vi "Tap Example.vi"() -> ()   [LabVIEW 2023, in "GettingStarted_Tap_148X_Host.lvlib"]
uses:
  GettingStarted_Tap_148X_Host.lvlib
  Acq/GettingStarted_Acq_148X_Host.lvlib
  <instrlib>/FlexRIO/API/Host/v1/NI FlexRIO API v1.lvlib
  Common/GettingStarted_Common_148X_Host.lvlib
  <vilib>/vision/Image Controls.llb/IMAQ Image.ctl
  Common/Types/Packet Table.ctl
  <vilib>/Utility/miscctls.llb/LVRowAndColumnUnsignedTypeDef.ctl
  <vilib>/rvi/interface/nirviCloseFPGA/nirviCloseFPGA.xnode
  <vilib>/FPGAPlugInAG/Dynamic/niLvFpga_Close_Dynamic.vi
  <instrlib>/FlexRIO/API/Host/v1/NI FlexRIO/API/Wait for PoC Safe to Disconnect Channels Array.vi
  <instrlib>/FlexRIO/CSI-2/v2/Common/Types/LLP Data Type.ctl
  <instrlib>/FlexRIO/CSI-2/v2/Common/NI CSI-2 API Common v2.lvlib
  <vilib>/userDefined/Silver/nirio_resource_slv.ctl
  Acq/Types/CSI-2 Data Source.ctl
  <instrlib>/FlexRIO/CSI-2/v2/FPGA/Types/Timestamp ID.ctl
  <instrlib>/FlexRIO/CSI-2/v2/FPGA/NI CSI-2 API FPGA v2.lvlib
  Common/Types/GPIO Filter.ctl
  <instrlib>/FlexRIO/CSI-2/v2/FPGA/Types/GPIO Bank.ctl
  FPGA/Common/Types/SerDes Identifier.ctl
  FPGA/Common/GettingStarted_Common_148X_FPGA.lvlib
  Common/Types/GPIO Route Direction.ctl
  Common/Types/GPIO Route Line.ctl
  Common/Types/GPIO Route Configuration.ctl
  <instrlib>/FlexRIO/CSI-2/v2/FPGA/Types/Display Parameters.ctl
  Common/Types/RAW Interpretation for Display.ctl
  Types/Serial Channel Tap Pair.ctl
  Types/Serial Channel Tap Configuration.ctl
panel:
  out "Acquisition Stopped":bool
  in  "Acquired Serial Input Channel Data":T1(tab)
  out "Source Rate (fps)(1st Display)":dbl
  out "Update Rate (fps)(1st Display)":dbl
  in  "Serial Channel (1st Display)":fxp<+,3,3>
  out "1st channel display":T2(plugin-control)
  out "Source Rate (fps)(2nd Display)":dbl
  out "Update Rate (fps)(2nd Display)":dbl
  out "2nd channel display":T2(plugin-control)
  in  "Serial Channel (2nd Display)":fxp<+,3,3>
  out "Acquired Packets (1st Channel)":T3
  out "Packets Logged (1st Channel)":i64
  out "Bytes Acquired (1st Channel)":i64 format="%#.6p"
  out "Acquired Packets (2nd Channel)":T3
  out "Packets Logged (2nd Channel)":i64
  out "Bytes Acquired (2nd Channel)":i64 format="%#.6p"
  out "I2C Timestamps":T3
  out "Error Parsing GPIO Timestamps":bool
  out "GPIO Timestamps Waveform":digitalwaveform[](graph)
  in  "Configuration":T4(tab)
  in  "Log Packets to Disk":bool
  in  "Display Acquired Images":bool=TRUE
  in  "RIO Device":T5
  in  "Bitfile Path":path
  in  "TDMS File Directory":path
  in  "Log I2C to Disk":bool
  in  "Log GPIO to Disk":bool
  in  "Logged Packets to Display":i64=1400
  in  "Channel Configurations":T6[](array[typedef])=[{"Serial Channel Tap Pair"={"input"="SI0", "output"="SO0"}, "FPGA Display Parameters"={"virtual channel"=0.0, "payload data type"=enum."RAW 12", "frame skip count"=0, "line skip count"=0, "pixel skip count"=0.0}, "RAW Display Parameters"={"Interpretation"=enum."Bayer", "Bayer Parameters"={"Pattern"=3, "Algorithm"=0, "Red Gain"=1.0, "Green Gain"=1.0, "Blue Gain"=1.0}}}] {"RAW Display Parameters"."Bayer Parameters"."Blue Gain" min=0.0 max=3.99 step=0.1 format="%_4g"; "RAW Display Parameters"."Bayer Parameters"."Green Gain" min=0.0 max=3.99 step=0.1 format="%_4g"; "RAW Display Parameters"."Bayer Parameters"."Red Gain" min=0.0 max=3.99 step=0.1 format="%_4g"; "RAW Display Parameters"."Bayer Parameters"."Algorithm" items=["Bilinear", "VNG"]; "RAW Display Parameters"."Bayer Parameters"."Pattern" items=["GB", "GR", "BG", "RG"]}
  in  "CSI-2 Data Source":T11=1 items=["Raw", "Corrected"]
  in  "Deserializer (Input) Configuration Script":path
  in  "Serializer (Output) Configuration Script":path
  in  "Continuous Acquisition":bool=TRUE
  in  "Acquisition Duration (s)":dbl=1.0 format="%#_13g"
  in  "Enable First and Last Packet Select":bool=TRUE
  in  "Stop Timeout (s)":dbl=1.0
  in  "First Packet Data Type Select":T9
  in  "Last Packet Data Type Select":T9=enum."Frame End"
  in  "Data Type Filter":T9[](array[typedef])
  in  "Virtual Channel Filter":fxp<+,4,4>[](array[numeric])
  in  "Invert Data Type Filter":bool
  in  "Invert Virtual Channel Filter":bool
  in  "Serial Input Active Lane Count":i32(ring)=4 items=["1 Lane"=1, "2 Lanes"=2, "4 Lanes"=4]
  out "Actual Serial Output Data Rate (bps)":dbl=-1.0 format="%#_6p"
  in  "Requested Serial Ouptut Data Rate (bps)":dbl=-1.0 format="%#_6p"
  in  "Serial Output Active Lane Count":i32(ring)=4 items=["1 Lane"=1, "2 Lanes"=2, "4 Lanes"=4]
  in  "Power Over Coax Source":i32(ring) items=["None", "Internal", "Auxiliary"]
  in  "Power Over Coax Sink":i32(ring) items=["None"=0, "Auxiliary"=2]
  in  "Serial Input Reference Clock Frequency (Hz)":dbl=25000000.0 format="%#_6p"
  in  "Serial Output Reference Clock Frequency (Hz)":dbl=25000000.0 format="%#_6p"
  in  "timestamp filter":T12[](array[typedef])
  in  "GPIO Bank Output Enable":T13
  in  "GPIO Routes":T14[](array[typedef]) {"Serial Channel" max=3 step=1}
  in  "GPIO Bank Select":T17
  in  "Update GPIO Output":bool
  in  "GPIO Bank Output":T13
  out "GPIO Bank Read":T13
  in  "GPIO to Display":T18[](array[typedef])
  out "Acquisition Duration (s)":dbl format="%.1f"
  out "Waiting for Sensor Setup":bool
  in  "Sensor Setup Complete":bool
  out "Power Over Coax Sink In Range":bool[](array[boolean])
  out "Acquisition In Progress":bool
  out "Power Over Coax Voltage (V)":dbl[](array[numeric]) format="%#.2pV"
  out "Power Over Coax Current (A)":dbl[](array[numeric]) format="%#.2pA"
  out "Power Over Coax Source In Range":bool[](array[boolean])
  in  "Stop Acquisition":bool
  out "Error Out":errorcluster
  # "Overview: Configure a tap acquisition for a CSI-2 sensor. Forward acquired CSI-2 data from the serial input channel to the paired serial output channel.\nBridge I2C communication between the paired serial output channel and serial input channel. Transfer the acquired data and timestamps to disk.\nInstructions: Visit https://ni.com/r/automotive-camera-module-ref for tutorials and reference material on using this example with the PXIe-148X."
  # "Configuration Settings"
  # "Data Output"
  # "* For additional packet viewing capability, use GettingStarted_Common_148X_Host.lvlib->TDMS File Viewer.vi"
  # "* For additional packet viewing capability, use GettingStarted_Common_148X_Host.lvlib->TDMS File Viewer.vi"
  # "Resource Configuration"
  # "Output Configuration"
  # "Channel Configuration"
  # "Acquisition Configuration"
  # "First and Last Packet Select Configuration"
  # "Packet Filter Configuration"
  # "Power Over Coax Configuration"
  # "Clocking Configuration"
  # "CSI-2 Output Configuration"
  # "Use -1 to request the default data rate"
  # "I2C Timestamp Configuration"
  # "The timestamp filters listed correspond to the I2C traffic for a specific serial channel:\n\nUser24 = SI0\nUser25 = SI1\nUser26 = SI2\nUser27 = SI3"
  # "GPIO Display Configuration"
  # "GPIO Bank Read / Write Configuration"
  # "GPIO Routing Configuration"
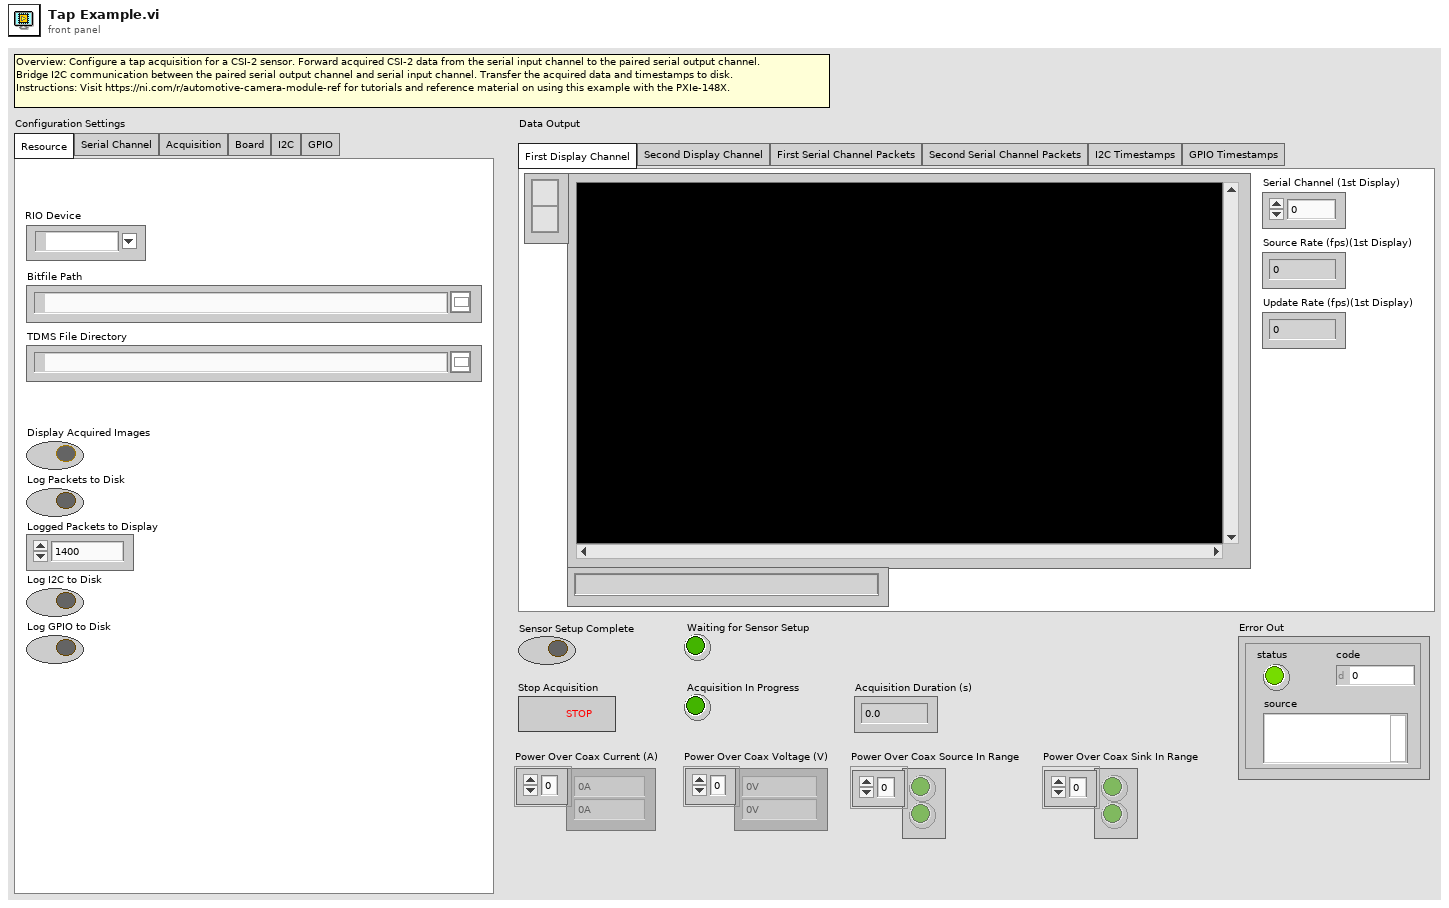
[diagram p1: front panel]
types:
  T1 = enum32{"First Display Channel", "Second Display Channel", "First Serial Channel Packets", "Second Serial Channel Packets", "I2C Timestamps", "GPIO Timestamps"}
  T2 = typedef "IMAQ Image.ctl" = refnum<image>
  T3 = typedef "GettingStarted_Common_148X_Host.lvlib/Packet Table.ctl" = string[][]
  T4 = enum32{"Resource", "Serial Channel", "Acquisition", "Board", "I2C", "GPIO"}
  T5 = typedef "nirio_resource_slv.ctl" = tag
  T6 = typedef "GettingStarted_Tap_148X_Host.lvlib/Serial Channel Tap Configuration.ctl" = cluster{"Serial Channel Tap Pair":T7, "FPGA Display Parameters":T8, "RAW Display Parameters":cluster{"Interpretation":T10, "Bayer Parameters":cluster{"Pattern":i32, "Algorithm":i32, "Red Gain":dbl, "Green Gain":dbl, "Blue Gain":dbl}}}
  T7 = typedef "GettingStarted_Tap_148X_Host.lvlib/Serial Channel Tap Pair.ctl" = cluster{"input":string, "output":string}
  T8 = typedef "NI CSI-2 API FPGA v2.lvlib/Display Parameters.ctl" = cluster{"virtual channel":fxp<+,4,4>, "payload data type":T9, "frame skip count":u16, "line skip count":u8, "pixel skip count":fxp<+,5,5>}
  T9 = typedef "NI CSI-2 API Common v2.lvlib/LLP Data Type.ctl" = enum8{"Frame Start", "Frame End", "Line Start", "Line End", "End of Transmission", "Reserved 0", "Reserved 1", "Reserved 2", "Generic Short Packet 1", "Generic Short Packet 2", "Generic Short Packet 3", "Generic Short Packet 4", "Generic Short Packet 5", "Generic Short Packet 6", "Generic Short Packet 7", "Generic Short Packet 8", "Null", "Blanking Data", "Embedded 8-bit non Image Data", "Generic Long Packet 1", "Generic Long Packet 2", "Generic Long Packet 3", "Generic Long Packet 4", "Reserved 3", "YUV420 8-bit", "YUV420 10-bit", "Legacy YUV420 8-bit", "Reserved 4", "YUV420 8-bit Chroma Shifted", "YUV420 10-bit Chroma Shifted", "YUV422 8-bit", "YUV422 10-bit", "RGB444", "RGB555", "RGB565", "RGB666", "RGB888", "Reserved 5", "Reserved 6", "RAW 24", "RAW 6", "RAW 7", "RAW 8", "RAW 10", "RAW 12", "RAW 14", "RAW 16", "RAW 20", "User Defined 8-bit Data 1", "User Defined 8-bit Data 2", "User Defined 8-bit Data 3", "User Defined 8-bit Data 4", "User Defined 8-bit Data 5", "User Defined 8-bit Data 6", "User Defined 8-bit Data 7", "User Defined 8-bit Data 8", "USL Command", "Reserved 7", "Reserved 8", "Reserved 9", "Reserved 10", "Reserved 11", "Reserved 12", "LRTE EPD Spacer"}
  T10 = typedef "GettingStarted_Common_148X_Host.lvlib/RAW Interpretation for Display.ctl" = enum16{"Grayscale", "Bayer", "RGB", "YUV422", "YUV420", "Legacy YUV420"}
  T11 = typedef "GettingStarted_Acq_148X_Host.lvlib/CSI-2 Data Source.ctl" = u16
  T12 = typedef "NI CSI-2 API FPGA v2.lvlib/Timestamp ID.ctl" = enum8{"SI0 LLP", "SI1 LLP", "SI2 LLP", "SI3 LLP", "SI4 LLP", "SI5 LLP", "SI6 LLP", "SI7 LLP", "SO0 LLP", "SO1 LLP", "SO2 LLP", "SO3 LLP", "SO4 LLP", "SO5 LLP", "SO6 LLP", "SO7 LLP", "Ser0 GPIO Bank", "Ser1 GPIO Bank", "Ser2 GPIO Bank", "Ser3 GPIO Bank", "Ser4 GPIO Bank", "Ser5 GPIO Bank", "Ser6 GPIO Bank", "Ser7 GPIO Bank", "Des0 GPIO Bank", "Des1 GPIO Bank", "Des2 GPIO Bank", "Des3 GPIO Bank", "Des4 GPIO Bank", "Des5 GPIO Bank", "Des6 GPIO Bank", "Des7 GPIO Bank", "User0", "User1", "User2", "User3", "User4", "User5", "User6", "User7", "User8", "User9", "User10", "User11", "User12", "User13", "User14", "User15", "User16", "User17", "User18", "User19", "User20", "User21", "User22", "User23", "User24", "User25", "User26", "User27", "User28", "User29", "User30", "User31"}
  T13 = typedef "NI CSI-2 API FPGA v2.lvlib/GPIO Bank.ctl" = cluster{"GPIO 0":bool, "GPIO 1":bool, "GPIO 2":bool, "GPIO 3":bool, "GPIO 4":bool, "GPIO 5":bool, "GPIO 6":bool, "GPIO 7":bool, "GPIO 8":bool, "GPIO 9":bool, "GPIO 10":bool}
  T14 = typedef "GettingStarted_Common_148X_Host.lvlib/GPIO Route Configuration.ctl" = cluster{"Direction":T15, "Serial Channel":u8, "Source":T16, "Destination":T16}
  T15 = typedef "GettingStarted_Common_148X_Host.lvlib/GPIO Route Direction.ctl" = enum8{"SO to SI", "SI to SO"}
  T16 = typedef "GettingStarted_Common_148X_Host.lvlib/GPIO Route Line.ctl" = enum16{"GPIO 0", "GPIO 1", "GPIO 2", "GPIO 3", "GPIO 4", "GPIO 5", "GPIO 6", "GPIO 7", "GPIO 8", "GPIO 9", "GPIO 10", "User"}
  T17 = typedef "GettingStarted_Common_148X_FPGA.lvlib/SerDes Identifier.ctl" = enum8{"None", "SI 0 Deserializer", "SI 1 Deserializer", "SI 2 Deserializer", "SI 3 Deserializer", "SI 4 Deserializer", "SI 5 Deserializer", "SI 6 Deserializer", "SI 7 Deserializer", "SO 0 Serializer", "SO 1 Serializer", "SO 2 Serializer", "SO 3 Serializer", "SO 4 Serializer", "SO 5 Serializer", "SO 6 Serializer", "SO 7 Serializer", "SI 0 SI 1 Deserializer", "SI 2 SI 3 Deserializer", "SI 4 SI 5 Deserializer", "SI 6 SI 7 Deserializer"}
  T18 = typedef "GettingStarted_Common_148X_Host.lvlib/GPIO Filter.ctl" = cluster{"GPIO Bank":T12, "GPIO Number":i32}
  T19 = typedef "LVRowAndColumnUnsignedTypeDef.ctl" = cluster{"Row":u32, "Column":u32}
  T20 = typedef "GettingStarted_Common_148X_Host.lvlib/Serial Channel Display Parameters.ctl" = cluster{"images":cluster{"grayscale":T2, "color":T2}, "RAW parameters":cluster{"interpretation":T10, "bayer parameters":cluster{"pattern":i32, "algorithm":i32, "red gain":dbl, "green gain":dbl, "blue gain":dbl}}}
  T21 = cluster{"Source Rate (fps)(1st Display)":refnum<vi>, "Update Rate (fps)(1st Display)":refnum<vi>}
  T22 = cluster{"Source Rate (fps)(2nd Display)":refnum<vi>, "Update Rate (fps)(2nd Display)":refnum<vi>}
  T23 = cluster{"Source Rate (fps)(2nd Display)":refnum<vi>, "Update Rate (fps)(2nd Display)":refnum<vi>}[]
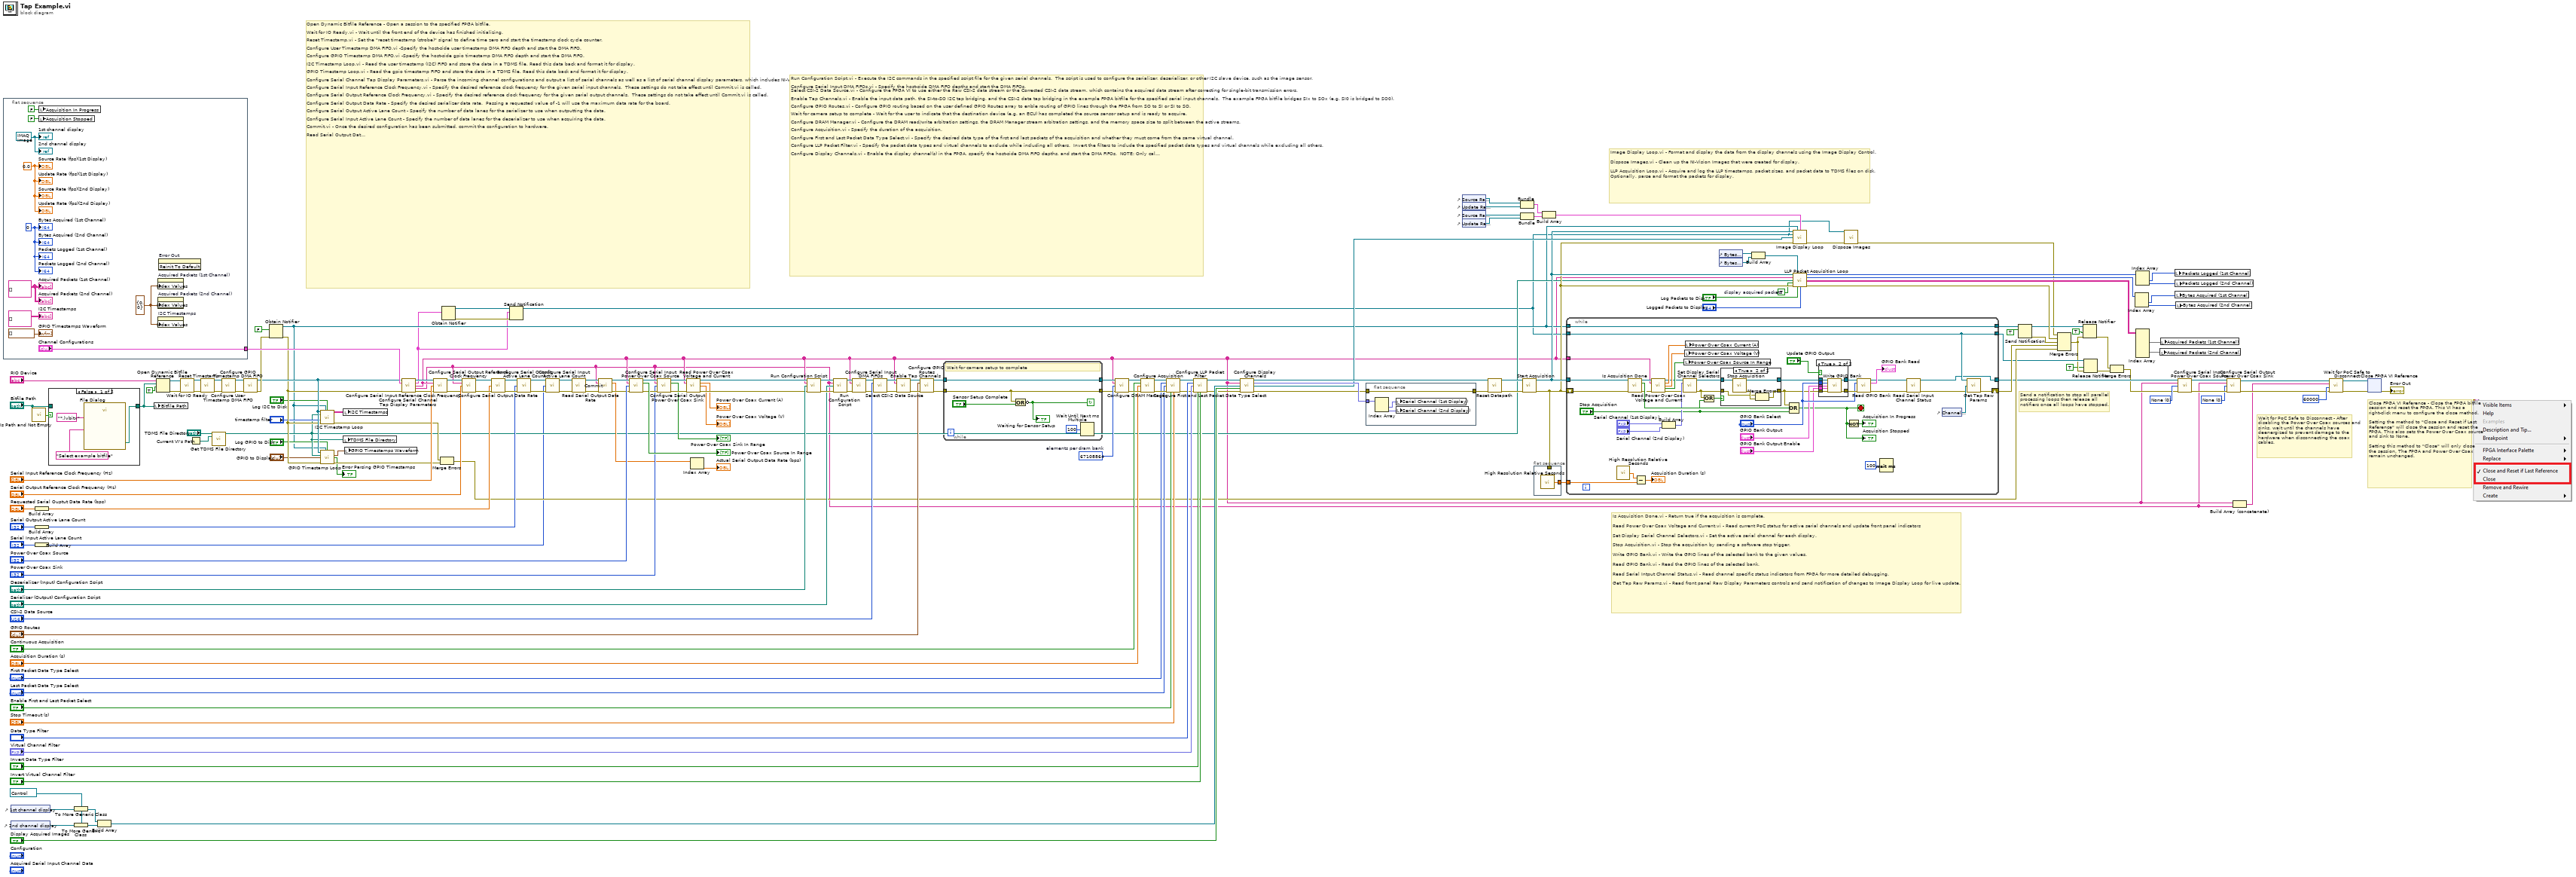
[diagram p0: block diagram]
diagram:
  w7 = 0 items=["None"=0, "Auxiliary"=2] ("power over coax sink")
  w9 = 0 items=["None", "Internal", "Auxiliary"] ("power over coax source")
  w35 = TRUE  # display acquired packets
  w125 = refnum<vi> refnum ("image display reference")
  w177 = u32 67108864  # elements per dram bank
  # "Wait for PoC Safe to Disconnect - After disabling the Power Over Coax sources and sinks, wait until the channels have deenergized to prevent damage to the hardware when disconnecting the coax cables."
  # "Close FPGA VI Reference - Close the FPGA bitfile session and reset the FPGA. This VI has a right-click menu to configure the close method. \n\nSetting the method to \"Close and Reset if Last Reference\" will close the session and reset the FPGA. This also sets the Power Over Coax source and sink to None.\n\nSetting this method to \"Close\" will only close the session. The FPGA and Power Over Coax remain unchanged."
  # "Send a notification to stop all parallel processing loops then release all notifiers once all loops have stopped."
  # "Is Acquisition Done.vi - Return true if the acquisition is complete.\n\nRead Power Over Coax Voltage and Current.vi - Read current PoC status for active serial channels and update front panel indicators \n\nSet Display Serial Channel Selectors.vi - Set the active serial channel for each display.\n\nStop Acquisition.vi - Stop the acquisition by sending a software stop trigger.\n\nWrite GPIO Bank.vi - Write the GPIO lines of the selected bank to the given values.\n\nRead GPIO Bank.vi - Read the GPIO lines of the selected bank.\n\nRead Serial Intput Channel Status.vi - Read channel specific status indicators from FPGA for more detailed debugging.\n\nGet Tap Raw Params.vi - Read front panel Raw Display Parameters controls and send notification of changes to Image Display Loop for live update."
  # "Image Display Loop.vi - Format and display the data from the display channels using the Image Display Control.  \n\nDispose Images.vi - Clean up the NI-Vision Images that were created for display.\n\nLLP Acquisition Loop.vi - Acquire and log the LLP timestamps, packet sizes, and packet data to TDMS files on disk.  Optionally, parse and format the packets for display."
  # "Run Configuration Script.vi - Execute the I2C commands in the specified script file for the given serial channels.  The script is used to configure the serializer, deserializer, or other I2C slave device, such as the image sensor.\n\nConfigure Serial Input DMA FIFOs.vi - Specify the host-side DMA FIFO depths and start the DMA FIFOs.\nSelect CSI-2 Data Source.vi - Configure the FPGA VI to use either the Raw CSI-2 data stream or the Corrected CSI-2 data stream, which contains the acquired data stream after correcting for single-bit transmission errors.\n\nEnable Tap Channels.vi - Enable the input data path, the SI-to-SO I2C tap bridging, and the CSI-2 data tap bridging in the example FPGA bitfile for the specified serial input channels.  The example FPGA bitfile bridges SIx to SOx (e.g. SI0 is bridged to SO0).\n\nConfigure GPIO Routes.vi - Configure GPIO routing based on the user defined GPIO Routes array to enble routing of GPIO lines through the FPGA from SO to SI or SI to SO. \n\nWait for camera setup to complete - Wait for the user to indicate that the destination device (e.g. an ECU) has completed the source sensor setup and is ready to acquire.\n\nConfigure DRAM Manager.vi - Configure the DRAM read/write arbitration settings, the DRAM Manager stream arbitration settings, and the memory space size to split between the active streams.\n\nConfigure Acquisition.vi - Specify the duration of the acquisition.\n\nConfigure First and Last Packet Data Type Select.vi - Specify the desired data type of the first and last packets of the acquisition and whether they must come from the same virtual channel.\n\nConfigure LLP Packet Filter.vi - Specify the packet data types and virtual channels to exclude while including all others.  Invert the filters to include the specified packet data types and virtual channels while excluding all others.\n\nConfigure Display Channels.vi - Enable the display channel(s) in the FPGA, specify the host-side DMA FIFO depths, and start the DMA FIFOs.  NOTE: Only called on Windows.  \n\nReset Datapath.vi - Issue the reset to all the VIs in the FPGA data path.\n\nStart Acquisition.vi - Start the acquisition by sending a software start trigger."
  # "Open Dynamic Bitfile Reference - Open a session to the specified FPGA bitfile.\n\nWait for IO Ready.vi - Wait until the front end of the device has finished initializing.\n\nReset Timestamp.vi - Set the \"reset timestamp (strobe)\" signal to define time zero and start the timestamp clock cycle counter.\n\nConfigure User Timestamp DMA FIFO.vi -Specify the host-side user timestamp DMA FIFO depth and start the DMA FIFO.\n\nConfigure GPIO Timestamp DMA FIFO.vi -Specify the host-side gpio timestamp DMA FIFO depth and start the DMA FIFO.\n\nI2C Timestamp Loop.vi - Read the user timestamp (I2C) FIFO and store the data in a TDMS file. Read this data back and format it for display.\n\nGPIO Timestamp Loop.vi - Read the gpio timestamp FIFO and store the data in a TDMS file. Read this data back and format it for display.\n\nConfigure Serial Channel Tap Display Parameters.vi - Parse the incoming channel configurations and output a list of serial channels as well as a list of serial channel display parameters, which includes NI-Vision Images and decoding parameters.\n\nConfigure Serial Input Reference Clock Frequency.vi - Specify the desired reference clock frequency for the given serial input channels.  These settings do not take effect until Commit.vi is called. \n\nConfigure Serial Output Reference Clock Frequency.vi - Specify the desired reference clock frequency for the given serial output channels.  These settings do not take effect until Commit.vi is called. \n\nConfigure Serial Output Data Rate - Specify the desired serializer data rate.  Passing a requested value of -1 will use the maximum data rate for the board.\n\nConfigure Serial Output Active Lane Count - Specify the number of data lanes for the serializer to use when outputting the data.\n\nConfigure Serial Input Active Lane Count - Specify the number of data lanes for the deserializer to use when acquiring the data.\n\nCommit.vi - Once the desired configuration has been submitted, commit the configuration to hardware.\n\nRead Serial Output Data Rate - Query the actual data rates of the serial output channels.  The driver might coerce the data rate to an achievable value\n\nConfigure Serial Input Power Over Coax Source.vi - Specify the source of the power that will be supplied to the devices via the coaxial cables attached to the given serial input channels.  These settings take effect in hardware immediately.\n\nConfigure Serial Output Power Over Coax Sink.vi - Specify whether to sink the power that will be supplied by the devices via the coaxial cables attached to the given serial output channels to the corresponding auxiliary power port.  These settings take effect in hardware immediately.\n\nRead Power Over Coax Voltage and Current.vi - Query the values of the voltage and current detected by the Power Over Coax circuitry of the given serial channels."
  n1 = flat-sequence {
    tunnel: ["Channel Configurations"] -> w102
    frame #0 {
      w180 = T19 {"Row"=0, "Column"=0} ("Index Values")
      w188 = T3 [] ("Acquired Packets (1st Channel)")
      w183 = 0 ("Number of Packets Acquired (1st Channel)")
      w189 = 0.0 ("display fps (2nd display)")
      w187 = T2 refnum ("first channel display")
      n2 = local write "Acquisition In Progress"(FALSE ("Acquisition In Progress")) -> ()
      n3 = local write "Acquisition Stopped"(FALSE ("Acquisition Stopped")) -> ()
      n4 = property on="Acquired Packets (1st Channel)" class="Tbl (strict)"("Index Values"=w180) -> ()  [unwired: 2 in, 2 out]
      n5 = property on="Acquired Packets (2nd Channel)" class="Tbl (strict)"("Index Values"=w180) -> ()  [unwired: 2 in, 2 out]
      n6 = property on="I2C Timestamps" class="Tbl (strict)"("Index Values"=w180) -> ()  [unwired: 2 in, 2 out]
      n7 = invoke on="Error Out" class="Clust (strict)" method="Reinit To Default"() -> ()  [unwired: 3 in, 3 out]
      "Update Rate (fps)(1st Display)" <- w189
      "Source Rate (fps)(1st Display)" <- w189
      "Update Rate (fps)(2nd Display)" <- w189
      "Source Rate (fps)(2nd Display)" <- w189
      "Packets Logged (1st Channel)" <- w183
      "Packets Logged (2nd Channel)" <- w183
      "Acquired Packets (1st Channel)" <- w188
      "Acquired Packets (2nd Channel)" <- w188
      "1st channel display" <- w187
      "2nd channel display" <- w187
      "GPIO Timestamps Waveform" <- digitalwaveform[] [] ("GPIO Timestamps Waveform")
      "I2C Timestamps" <- T3 [] ("I2C Timestamps 2")
      "Bytes Acquired (2nd Channel)" <- w183
      "Bytes Acquired (1st Channel)" <- w183
    }
  }
  n8 = control-ref of="1st channel display"() -> (w121:refnum<vi>)
  n9 = control-ref of="2nd channel display"() -> (w122:refnum<vi>)
  n10 = call <vilib>:"Is Path and Not Empty.vi"("path"="Bitfile Path") -> ("Is Path and Not Empty?"=w166:bool)  [unwired: 4 in]
  n11 = Build Array("Requested Serial Ouptut Data Rate (bps)") -> (w56:dbl[])
  n12 = Build Array("Serial Output Active Lane Count") -> (w55:i32[])
  n13 = Build Array("Serial Input Active Lane Count") -> (w26:i32[])
  n14 = case shown="False" w166 {
    tunnel: "Bitfile Path" -> [_ w193]
    tunnel: [w191 w193] -> w165
    frame False {
      n15 = call "File Dialog"("prompt"="Select example bitfile", "pattern (all files)"="*.lvbitx") -> ("selected path"=w191:path)  [unwired: 10 in, 3 out]
    }
    frame True {
    }
  }
  n16 = To More Generic Class(target class=w125, reference=w121) -> (generic class reference=w124:refnum<vi>)
  n17 = To More Generic Class(target class=w125, reference=w122) -> (generic class reference=w123:refnum<vi>)
  n18 = Build Array(w124, w123) -> (w99:refnum<vi>[])
  n19 = local write "Bitfile Path"(w165) -> ()
  n20 = Open Dynamic Bitfile Reference(0:"RIO Device", 1:w165, 2:TRUE ("Run When Loaded")) -> (5:w163:refnum<k20>, 8:w164:errorcluster)  [unwired: 2 in]
  n21 = call <instrlib>:"Wait for IO Ready.vi"("fpga interface in"=w163, "error in"=w164) -> ("fpga interface out"=w77:refnum<k20>, "error out"=w78:errorcluster)  [unwired: 10 in, 2 out]
  n22 = Current VI's Path() -> (path=w120:path)
  n23 = call "Reset Timestamp.vi"("fpga interface in"=w77, "error in (no error)"=w78) -> ("fpga interface out"=w54:refnum<k20>, "error out"=w53:errorcluster)  [unwired: 12 in]
  n24 = call "Get TDMS File Directory.vi"("tdms file directory in"="TDMS File Directory", "calling vi path"=w120) -> ("tdms file directory out"=w41:path)  [unwired: 13 in]
  n25 = call "Configure User Timestamp DMA FIFO.vi"("fpga interface in"=w54, "error in (no error)"=w53) -> ("fpga interface out"=w52:refnum<k20>, "error out"=w51:errorcluster)  [unwired: 12 in]
  n26 = call "Configure GPIO Timestamp DMA FIFO.vi"("fpga interface in"=w52, "error in (no error)"=w51) -> ("fpga interface out"=w48:refnum<k20>, "error out"=w50:errorcluster)  [unwired: 12 in]
  n27 = Obtain Notifier(notification data type=FALSE ("result"), error in (no error)=w50) -> (notifier out=w25:refnum<notifier>, error out=w47:errorcluster)  [unwired: 2 in, 1 out]
  n28 = call "I2C Timestamp Loop.vi"("fpga interface in"=w48, "'stop' notifier"=w25, "log i2c to disk"="Log I2C to Disk", "tdms file directory"=w41, "timestamp filter"="timestamp filter", "error in (no error)"=w47) -> ("i2c data"=w40:string[][], "error out"=w46:errorcluster)  [unwired: 8 in]
  n29 = call "GPIO Timestamp Loop.vi"("fpga interface in"=w48, "'stop' notifier"=w25, "log gpio to disk"="Log GPIO to Disk", "tdms file directory"=w41, "gpio to display"="GPIO to Display", "error in (no error)"=w47) -> ("gpio timestamps waveform"=w39:digitalwaveform[], "error parsing gpio timestamps"=→"Error Parsing GPIO Timestamps":bool, "error out"=w45:errorcluster)  [unwired: 7 in]
  n30 = local write "I2C Timestamps"(w40) -> ()
  n31 = local write "TDMS File Directory"(w41) -> ()
  n32 = local write "GPIO Timestamps Waveform"(w39) -> ()
  n33 = call "Configure Serial Channel Tap Display Parameters.vi"("fpga interface in"=w48, "serial channel configurations"=w102, "error in (no error)"=w47) -> ("fpga interface out"=w103:refnum<k20>, "serial channel display parameters"=w22:T20[], "serial input channels"=w3:string[], "serial output channels"=w2:string[], "error out"=w104:errorcluster)  [unwired: 8 in]
  n34 = call "Configure Serial Input Reference Clock Frequency.vi"("fpga interface in"=w103, "serial input channels"=w3, "serial input reference clock frequency (Hz)"="Serial Input Reference Clock Frequency (Hz)", "error in (no error)"=w104) -> ("fpga interface out"=w153:refnum<k20>, "error out"=w152:errorcluster)  [unwired: 10 in]
  n35 = Merge Errors(w46, w45) -> (w32:errorcluster)
  n36 = Obtain Notifier(notification data type=w22) -> (notifier out=w24:refnum<notifier>, error out=w23:errorcluster)  [unwired: 3 in, 1 out]
  n37 = call "Configure Serial Output Reference Clock Frequency.vi"("fpga interface in"=w153, "serial output channels"=w2, "serial output reference clock frequency (Hz)"="Serial Output Reference Clock Frequency (Hz)", "error in (no error)"=w152) -> ("fpga interface out"=w68:refnum<k20>, "error out"=w67:errorcluster)  [unwired: 10 in]
  n38 = call "Configure Serial Output Data Rate.vi"("fpga interface in"=w68, "serial output data rates"=w56, "error in (no error)"=w67) -> ("fpga interface out"=w65:refnum<k20>, "error out"=w66:errorcluster)  [unwired: 11 in]
  n39 = Send Notification(notification=w22, notifier=w24, error in (no error)=w23) -> (notifier out=w21:refnum<notifier>)  [unwired: 1 out]
  n40 = call "Configure Serial Output Active Lane Count.vi"("fpga interface in"=w65, "serial output active lane counts"=w55, "error in (no error)"=w66) -> ("fpga interface out"=w31:refnum<k20>, "error out"=w30:errorcluster)  [unwired: 11 in]
  n41 = call "Configure Serial Input Active Lane Count.vi"("fpga interface in"=w31, "serial input active lane counts"=w26, "error in (no error)"=w30) -> ("fpga interface out"=w29:refnum<k20>, "error out"=w28:errorcluster)  [unwired: 11 in]
  n42 = call <instrlib>:"Commit.vi"("fpga interface in"=w29, "error in"=w28) -> ("fpga interface out"=w63:refnum<k20>, "error out"=w64:errorcluster)  [unwired: 12 in]
  n43 = call "Read Serial Output Data Rate.vi"("fpga interface in"=w63, "serial output channels"=w2, "error in (no error)"=w64) -> ("fpga interface out"=w61:refnum<k20>, "serial output data rates (bps)"=w59:dbl[], "error out"=w62:errorcluster)  [unwired: 10 in]
  n44 = call "Configure Serial Input Power Over Coax Source.vi"("fpga interface in"=w61, "serial input channels"=w3, "power over coax source"="Power Over Coax Source", "error in (no error)"=w62) -> ("fpga interface out"=w146:refnum<k20>, "power over coax source in range"=→"Power Over Coax Source In Range":bool[], "error out"=w143:errorcluster)  [unwired: 9 in]
  n45 = call "Configure Serial Output Power Over Coax Sink.vi"("fpga interface in"=w146, "serial output channels"=w2, "power over coax sink"="Power Over Coax Sink", "error in (no error)"=w143) -> ("fpga interface out"=w145:refnum<k20>, "power over coax sink in range"=→"Power Over Coax Sink In Range":bool[], "error out"=w144:errorcluster)  [unwired: 9 in]
  n46 = call "Read Power Over Coax Voltage and Current.vi"("fpga interface in"=w145, "serial channels"=w3, "error in (no error)"=w144) -> ("fpga interface out"=w160:refnum<k20>, "current (A)"=→"Power Over Coax Current (A)":dbl[], "voltage (V)"=→"Power Over Coax Voltage (V)":dbl[], "error out"=w161:errorcluster)  [unwired: 8 in, 1 out]
  n47 = Index Array(array=w59) -> (element=→"Actual Serial Output Data Rate (bps)":dbl)  [unwired: 1 in]
  n48 = call "Run Configuration Script.vi"("fpga interface in"=w160, "serial channels"=w3, "configuration script"="Deserializer (Input) Configuration Script", "error in (no error)"=w161) -> ("fpga interface out"=w151:refnum<k20>, "error out"=w148:errorcluster)  [unwired: 10 in]
  n49 = call "Run Configuration Script.vi"("fpga interface in"=w151, "serial channels"=w2, "configuration script"="Serializer (Output) Configuration Script", "error in (no error)"=w148) -> ("fpga interface out"=w150:refnum<k20>, "error out"=w149:errorcluster)  [unwired: 10 in]
  n50 = call "Configure Serial Input DMA FIFOs.vi"("fpga interface in"=w150, "serial channels"=w3, "error in (no error)"=w149) -> ("fpga interface out"=w137:refnum<k20>, "error out"=w136:errorcluster)  [unwired: 11 in]
  n51 = call "Select CSI-2 Data Source.vi"("fpga interface in"=w137, "csi-2 data source"="CSI-2 Data Source", "error in (no error)"=w136) -> ("fpga interface out"=w134:refnum<k20>, "error out"=w135:errorcluster)  [unwired: 11 in]
  n52 = call "Enable Tap Channels.vi"("fpga interface in"=w134, "serial input channels"=w3, "error in (no error)"=w135) -> ("fpga interface out"=w82:refnum<k20>, "error out"=w83:errorcluster)  [unwired: 11 in]
  n53 = call "Configure GPIO Routes.vi"("fpga interface in"=w82, "gpio routes"="GPIO Routes", "error in (no error)"=w83) -> ("fpga interface out"=w81:refnum<k20>, "error out"=w80:errorcluster)  [unwired: 11 in]
  n54 = while {
    tunnel: w80 -> [w198]
    tunnel: [w198] -> w140
    tunnel: w81 -> [w196]
    tunnel: [w196] -> w139
    stop <- w194 continue-if-true
    # "Wait for camera setup to complete"
    n55 = Compound Arithmetic op=OR(w198, "Sensor Setup Complete") -> (invert w194:bool)
    "Waiting for Sensor Setup" <- w194
    n56 = Wait Until Next ms Multiple(millisecond multiple=u32 100) -> ()  [unwired: 1 out]
  }
  n57 = call "Configure DRAM Manager.vi"("fpga interface in"=w139, "serial channels"=w3, "elements per dram bank"=w177, "error in (no error)"=w140) -> ("fpga interface out"=w176:refnum<k20>, "error out"=w178:errorcluster)  [unwired: 10 in]
  n58 = call "Configure Acquisition.vi"("fpga interface in"=w176, "continuous acquisition (T)"="Continuous Acquisition", "acquisition duration (s)"="Acquisition Duration (s)", "error in (no error)"=w178) -> ("fpga interface out"=w130:refnum<k20>, "error out"=w133:errorcluster)  [unwired: 10 in]
  n59 = call "Configure First and Last Packet Data Type Select.vi"("fpga interface in"=w130, "first packet data type select"="First Packet Data Type Select", "last packet data type select"="Last Packet Data Type Select", "error in (no error)"=w133, "enable first and last packet select"="Enable First and Last Packet Select", "stop timeout (s)"="Stop Timeout (s)") -> ("fpga interface out"=w131:refnum<k20>, "error out"=w132:errorcluster)  [unwired: 8 in]
  n60 = call "Configure LLP Packet Filter.vi"("fpga interface in"=w131, "data type filter"="Data Type Filter", "virtual channel filter"="Virtual Channel Filter", "error in (no error)"=w132, "invert data type filter"="Invert Data Type Filter", "invert virtual channel filter"="Invert Virtual Channel Filter") -> ("fpga interface out"=w100:refnum<k20>, "error out"=w97:errorcluster)  [unwired: 8 in]
  n61 = call "Configure Display Channels.vi"("fpga interface in"=w100, "serial channels"=w3, "display references in"=w99, "enable image display"="Display Acquired Images", "error in (no error)"=w97) -> ("fpga interface out"=w96:refnum<k20>, "display serial channels"=w95:fxp<+,3,3>[], "display references out"=w92:refnum<vi>[], "error out"=w94:errorcluster)  [unwired: 7 in]
  n62 = flat-sequence {
    tunnel: w95 -> [w200]
    tunnel: w94 -> [w199]
    tunnel: [w199] -> w126
    frame #0 {
      n63 = Index Array(array=w200) -> (element #1=w202:fxp<+,3,3>, element #2=w201:fxp<+,3,3>)  [unwired: 2 in]
      n64 = local write "Serial Channel (1st Display)"(w202) -> ()
      n65 = local write "Serial Channel (2nd Display)"(w201) -> ()
    }
  }
  n66 = control-ref of="Source Rate (fps)(1st Display)"() -> (w107:refnum<vi>)
  n67 = control-ref of="Update Rate (fps)(1st Display)"() -> (w108:refnum<vi>)
  n68 = control-ref of="Source Rate (fps)(2nd Display)"() -> (w105:refnum<vi>)
  n69 = control-ref of="Update Rate (fps)(2nd Display)"() -> (w106:refnum<vi>)
  n70 = call "Reset Datapath.vi"("fpga interface in"=w96, "error in (no error)"=w126) -> ("fpga interface out"=w175:refnum<k20>, "error out"=w49:errorcluster)  [unwired: 12 in]
  n71 = Bundle("Source Rate (fps)(1st Display)"=w107, "Update Rate (fps)(1st Display)"=w108) -> (w113:T21)  [unwired: 1 in]
  n72 = Bundle("Source Rate (fps)(2nd Display)"=w105, "Update Rate (fps)(2nd Display)"=w106) -> (w112:T22)  [unwired: 1 in]
  n73 = call "Start Acquisition.vi"("fpga interface in"=w175, "error in (no error)"=w49) -> ("fpga interface out"=w90:refnum<k20>, "error out"=w88:errorcluster)  [unwired: 12 in]
  n74 = flat-sequence {
    tunnel: [w203] -> w101
    tunnel: w88 -> [_]
    frame #0 {
      n75 = call <vilib>:"High Resolution Relative Seconds.vi"() -> ("relative seconds"=w203:dbl)
    }
  }
  n76 = Build Array(w113, w112) -> (w91:T23)
  n77 = while {
    shift-right: [w210] -> w33
    shift-left: w88 -> [w230]
    tunnel: w90 -> [w231]
    tunnel: [w204] -> w10
    tunnel: w3 -> [w240]
    tunnel: w101 -> [w235]
    tunnel: w25 -> [w211]
    tunnel: [w211] -> w70
    tunnel: w21 -> [w208]
    tunnel: [w208] -> w20
    stop <- w212 stop-if-true
    n78 = call <vilib>:"High Resolution Relative Seconds.vi"() -> ("relative seconds"=w236:dbl)
    n79 = call "Is Acquisition Done.vi"("fpga interface in"=w231, "error in (no error)"=w230) -> ("fpga interface out"=w241:refnum<k20>, "acquisition done"=w244:bool, "error out"=w242:errorcluster)  [unwired: 11 in]
    n80 = Subtract(x=w236, y=w235) -> (x-y=→"Acquisition Duration (s)":dbl)
    n81 = call "Read Power Over Coax Voltage and Current.vi"("fpga interface in"=w241, "serial channels"=w240, "error in (no error)"=w242) -> ("fpga interface out"=w233:refnum<k20>, "current (A)"=w239:dbl[], "voltage (V)"=w237:dbl[], "in range"=w238:bool[], "error out"=w232:errorcluster)  [unwired: 8 in]
    n82 = Build Array("Serial Channel (1st Display)", "Serial Channel (2nd Display)") -> (w234:fxp<+,3,3>[])
    n83 = call "Set Display Serial Channel Selectors.vi"("fpga interface in"=w233, "display serial channel selectors"=w234, "error in (no error)"=w232) -> ("fpga interface out"=w229:refnum<k20>, "error out"=w228:errorcluster)  [unwired: 11 in]
    n84 = local write "Power Over Coax Source In Range"(w238) -> ()
    n85 = local write "Power Over Coax Voltage (V)"(w237) -> ()
    n86 = local write "Power Over Coax Current (A)"(w239) -> ()
    n87 = Compound Arithmetic op=OR(w228, "Stop Acquisition") -> (w227:bool)
    n88 = case shown="True" w227 {
      tunnel: [w255 w257] -> w214
      tunnel: w228 -> [w255 w256]
      tunnel: [w254 w259] -> w218
      tunnel: w229 -> [w254 w258]
      frame False {
      }
      frame True {
        n89 = call "Stop Acquisition.vi"("fpga interface in"=w258) -> ("fpga interface out"=w259:refnum<k20>, "error out"=w260:errorcluster)  [unwired: 13 in]
        n90 = Merge Errors(w256, w260) -> (w257:errorcluster)
      }
    }
    n91 = Compound Arithmetic op=OR(w214, w244, "Stop Acquisition") -> (w212:bool)
    "Acquisition Stopped" <- w212
    n92 = case shown="True" "Update GPIO Output" {
      tunnel: w218 -> [w246 w253]
      tunnel: w214 -> [w245 w252]
      tunnel: "GPIO Bank Output" -> [_ w251]
      tunnel: [w246 w250] -> w221
      tunnel: [w245 w249] -> w220
      tunnel: "GPIO Bank Select" -> [_ w248]
      tunnel: "GPIO Bank Output Enable" -> [_ w247]
      frame False {
      }
      frame True {
        n93 = call "Write GPIO Bank.vi"("fpga interface in"=w253, "gpio bank select"=w248, "gpio bank output"=w251, "gpio bank output enable"=w247, "error in (no error)"=w252) -> ("fpga interface out"=w250:refnum<k20>, "error out"=w249:errorcluster)  [unwired: 9 in]
      }
    }
    n94 = Not(x=w212) -> (.not. x?=→"Acquisition In Progress":bool)
    n95 = call "Read GPIO Bank.vi"("fpga interface in"=w221, "gpio bank select"="GPIO Bank Select", "error in (no error)"=w220) -> ("fpga interface out"=w207:refnum<k20>, "gpio bank output"=→"GPIO Bank Read":T13, "error out"=w206:errorcluster)  [unwired: 10 in]
    n96 = Wait (ms)(milliseconds to wait=u32 100) -> ()  [unwired: 1 out]
    n97 = call "Read Serial Input Channel Status.vi"("fpga interface in"=w207, "error in (no error)"=w206) -> ("fpga interface out"=w204:refnum<k20>, "error out"=w205:errorcluster)  [unwired: 11 in, 1 out]
    n98 = control-ref of="Channel Configurations"() -> (w209:refnum<vi>)
    n99 = call "Get Tap Raw Params.vi"("raw display notifier"=w208, "Channel Configurations"=w209, "error in (no error)"=w205) -> ("error out"=w210:errorcluster)  [unwired: 12 in]
  }
  n100 = control-ref of="Bytes Acquired (1st Channel)"() -> (w110:refnum<vi>)
  n101 = control-ref of="Bytes Acquired (2nd Channel)"() -> (w109:refnum<vi>)
  n102 = Build Array(w110, w109) -> (w119:refnum<vi>[])
  n103 = call "Image Display Loop.vi"("fpga interface in"=w90, "'stop' notifier"=w25, "rate references"=w91, "raw display notifier"=w21, "display references"=w92, "error in (no error)"=w88) -> ("error out"=w93:errorcluster)  [unwired: 9 in]
  n104 = call "LLP Packet Acquisition Loop.vi"("fpga interface in"=w90, "bytes acquired references"=w119, "Serial Channels"=w3, "tdms file directory"=w41, "display acquired packets"=w35, "error in"=w88, "log to disk"="Log Packets to Disk", "num packets to read"="Logged Packets to Display") -> ("number of packets acquired"=w118:i64[], "number of bytes acquired"=w85:i64[], "display data"=w84:string[][][], "error out"=w74:errorcluster)  [unwired: 4 in]
  n105 = call "Dispose Images.vi"("raw display notifier"=w21, "error in (no error)"=w93) -> ("error out"=w44:errorcluster)  [unwired: 13 in]
  n106 = Send Notification(notification=TRUE, notifier=w70) -> (notifier out=w72:refnum<notifier>, error out=w73:errorcluster)  [unwired: 1 in]
  n107 = Merge Errors(w44, w74, w73, w33, w32) -> (w19:errorcluster)
  n108 = Release Notifier(notifier=w72, force destroy? (F)=TRUE, error in (no error)=w19) -> (error out=w17:errorcluster)  [unwired: 2 out]
  n109 = Release Notifier(notifier=w20, force destroy? (F)=TRUE, error in (no error)=w19) -> (error out=w16:errorcluster)  [unwired: 2 out]
  n110 = Merge Errors(w17, w16) -> (w8:errorcluster)
  n111 = Index Array(array=w85) -> (element #1=w86:i64, element #2=w87:i64)  [unwired: 2 in]
  n112 = Index Array(array=w118) -> (element #1=w117:i64, element #2=w116:i64)  [unwired: 2 in]
  n113 = Index Array(array=w84) -> (element #1=w115:string[][], element #2=w114:string[][])  [unwired: 6 in]
  n114 = local write "Acquired Packets (2nd Channel)"(w114) -> ()
  n115 = local write "Acquired Packets (1st Channel)"(w115) -> ()
  n116 = local write "Packets Logged (1st Channel)"(w117) -> ()
  n117 = local write "Packets Logged (2nd Channel)"(w116) -> ()
  n118 = local write "Bytes Acquired (1st Channel)"(w86) -> ()
  n119 = local write "Bytes Acquired (2nd Channel)"(w87) -> ()
  n120 = call "Configure Serial Input Power Over Coax Source.vi"("fpga interface in"=w10, "serial input channels"=w3, "power over coax source"=w9, "error in (no error)"=w8) -> ("fpga interface out"=w6:refnum<k20>, "error out"=w13:errorcluster)  [unwired: 9 in, 1 out]
  n121 = call "Configure Serial Output Power Over Coax Sink.vi"("fpga interface in"=w6, "serial output channels"=w2, "power over coax sink"=w7, "error in (no error)"=w13) -> ("fpga interface out"=w5:refnum<k20>, "error out"=w12:errorcluster)  [unwired: 9 in, 1 out]
  n122 = Build Array (concatenate)(w3, w2) -> (w1:string[])
  n123 = call-poly <instrlib>:"Wait for PoC Safe to Disconnect.vi"("error in"=w12, "Timeout (ms)"=60000 ("Wait for Safe to Disconnect Timeout (ms)"), "Channels"=w1, "fpga interface in"=w5) -> ("error out"=w14:errorcluster, "fpga interface out"=w4:refnum<k20>)  [unwired: 6 in]
  n124 = xnode ("Close FPGA VI Reference")("FPGA VI Reference In"=w4, "error in"=w14) -> ("error out"=→"Error Out":errorcluster)
